vi "Set_Names_ID_Experiments.vi"(8 "error in (no error)":errorcluster, 11 "DB in":refnum<class "DB.lvclass">) -> (0 "error out":errorcluster, 3 "DB out":refnum<class "DB.lvclass">)   [LabVIEW 2015, in "DB.lvclass"]
uses:
  DB.lvclass
  DB.lvclass/DB.ctl
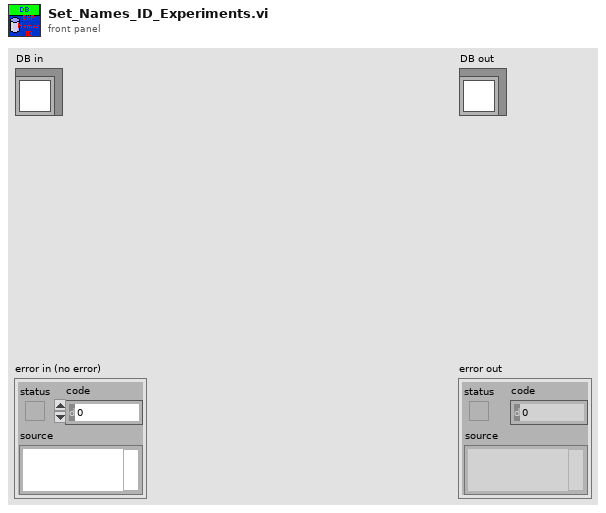
[diagram p1: front panel]
types:
  T1 = typedef "DB.lvclass/Def_fix_sql_param.ctl" = cluster{"Fix Project":bool, "Fix Sample":bool, "Fix Exp Date":bool, "Fix User":bool}
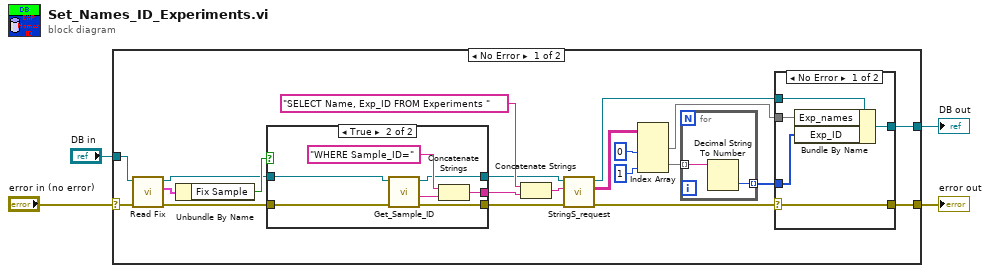
[diagram p0: block diagram]
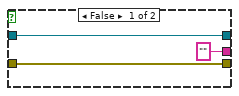
[diagram p2: hidden frame]
diagram:
  n1 = case shown="No Error" "error in (no error)" {
    selector: "error in (no error)" -> [w8 w46]
    tunnel: [w16 w46] -> w3
    tunnel: [w17 w45] -> w1
    tunnel: "DB in" -> [w9 w45]
    frame No Error {
      n2 = call "Read Fix.vi"("error in (no error)"=w8, "DB in"=w9) -> ("error out"=w10:errorcluster, "Fix"=w15:T1, "DB out"=w11:refnum<class "DB.lvclass">)  [unwired: 7 in]
      n3 = Unbundle By Name(w15) -> ("Fix Sample"=w14:bool)
      n4 = case shown="True" w14 {
        tunnel: ["" w34] -> w13
        tunnel: w11 -> [w28 w33]
        tunnel: [w28 w31] -> w6
        tunnel: w10 -> [w27 w30]
        tunnel: [w27 w29] -> w5
        frame False {
        }
        frame True {
          n5 = call "Get_Sample_ID.vi"("error in (no error)"=w30, "DB in"=w33) -> ("error out"=w29:errorcluster, "Sample_ID"=w32:string, "DB out"=w31:refnum<class "DB.lvclass">)  [unwired: 6 in, 1 out]
          n6 = Concatenate Strings("WHERE Sample_ID=", w32) -> (w34:string)
        }
      }
      n7 = Concatenate Strings("SELECT Name, Exp_ID FROM Experiments " ("SQL"), w13) -> (w7:string)
      n8 = call-dynamic "StringS_request.vi"("error in (no error)"=w5, "SQL request"=w7, "DB in"=w6) -> ("error out"=w23:errorcluster, "Result Set"=w21:string[][], "DB out"=w25:refnum<class "DB.lvclass">)  [unwired: 5 in, 1 out]
      n9 = Index Array(array=w21, index (col) #1=0 ("disabled index (col)"), index (col) #2=1 ("index (col)")) -> (element #1=w24:string[], element #2=w20:string[])  [unwired: 2 in]
      n10 = for {
        tunnel: w20 -> [w44] mode=indexing
        tunnel: [w43] -> w22 mode=indexing
        n11 = Decimal String To Number(string=w44) -> (number=w43:i32)  [unwired: 2 in, 1 out]
      }
      n12 = case shown="No Error" w23 {
        selector: w23 -> [w36 w41]
        tunnel: w25 -> [w40 w42]
        tunnel: [w39 w42] -> w17
        tunnel: w22 -> [w38 _]
        tunnel: w24 -> [w37 _]
        tunnel: [w36 w41] -> w16
        frame No Error {
          n13 = Bundle By Name(cluster=w40, "Exp_names"=w37, "Exp_ID"=w38) -> (w39:refnum<class "DB.lvclass">)
        }
        frame Error {
        }
      }
    }
    frame Error {
    }
  }
  "error out" <- w3
  "DB out" <- w1
